vi "Set Debug Mode.vi"(8 "error in (no error)":errorcluster, 10 "debug":bool, 11 "path-with-auto-complete in":refnum<class "path-with-auto-complete.lvclass">) -> (0 "error out":errorcluster, 3 "path-with-auto-complete out":refnum<class "path-with-auto-complete.lvclass">)   [LabVIEW 2020, in "path-with-auto-complete.lvclass"]
doc: "The <b>Load State Data VI</b> is a dynamic dispatch VI that must be overwritten in every QControl Class that uses the State Data. If used it must <b>Call Parent Method</b>. This recursively loads the Data Value Reference to the data space for the QControl Class up the inheritance hierarchy that uses the Data Value Reference.\n<b> </b> <b> </b>\n©2016 Q Software Innovations, LLC (QSI)\nwritten by Quentin Alldredge\nproduced in LabVIEW 2015\n\nsupport@qsoftwareinnovations.com\nwww.qsoftwareinnovations.com\n\nAll rights reserved.\n\nRedistribution and use in source and binary forms, with or without modification, are permitted provided that the following conditions are met:\n\n * Redistributions of source code must retain the above copyright notice, this list of conditions and the following disclaimer.\n * Redistributions in binary form must reproduce the above copyright notice, this list of conditions and the following disclaimer in the documentation and/or other materials provided with the distribution.\n * Neither the name of Q Software Innovations, LLC. nor the names of its contributors may be used to endorse or promote products derived from this software without specific prior written permission.\n\nTHIS SOFTWARE IS PROVIDED BY THE COPYRIGHT HOLDERS AND CONTRIBUTORS \"AS IS\" AND ANY EXPRESS OR IMPLIED WARRANTIES, INCLUDING, BUT NOT LIMITED TO, THE IMPLIED WARRANTIES OF MERCHANTABILITY AND FITNESS FOR A PARTICULAR PURPOSE ARE DISCLAIMED. IN NO EVENT SHALL THE COPYRIGHT OWNER OR CONTRIBUTORS BE LIABLE FOR ANY DIRECT, INDIRECT, INCIDENTAL, SPECIAL, EXEMPLARY, OR CONSEQUENTIAL DAMAGES (INCLUDING, BUT NOT LIMITED TO, PROCUREMENT OF SUBSTITUTE GOODS OR SERVICES; LOSS OF USE, DATA, OR PROFITS; OR BUSINESS INTERRUPTION) HOWEVER CAUSED AND ON ANY THEORY OF LIABILITY, WHETHER IN CONTRACT, STRICT LIABILITY, OR TORT (INCLUDING NEGLIGENCE OR OTHERWISE) ARISING IN ANY WAY OUT OF THE USE OF THIS SOFTWARE, EVEN IF ADVISED OF THE POSSIBILITY OF SUCH DAMAGE."
uses:
  path-with-auto-complete.lvclass
  path-with-auto-complete.lvclass/path-with-auto-complete.ctl
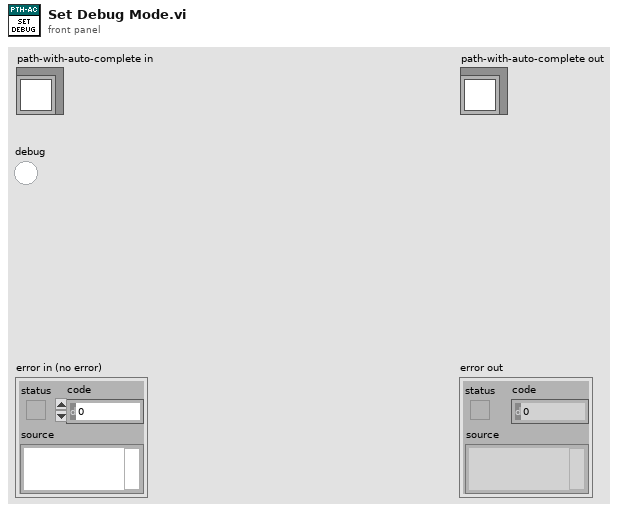
[diagram p1: front panel]
types:
  T1 = typedef "path-with-auto-complete.lvclass/State Data.ctl" = cluster{"Data":bool, "debug":bool, "mouse-down":bool, "has-focus":bool}
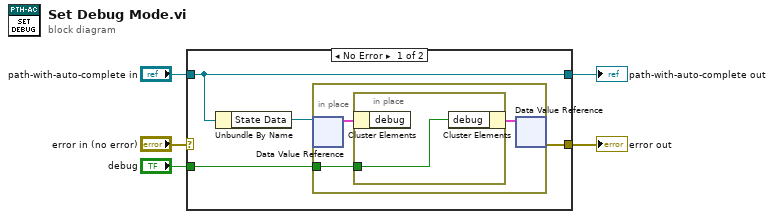
[diagram p0: block diagram]
diagram:
  n1 = case shown="No Error" "error in (no error)" {
    selector: "error in (no error)" -> [_ w15]
    tunnel: [w9 w15] -> w4
    tunnel: [w8 w14] -> w3
    tunnel: "path-with-auto-complete in" -> [w8 w14]
    tunnel: "debug" -> [w6 _]
    frame No Error {
      n2 = Unbundle By Name(w8) -> ("State Data"=w7:refnum<data-value>)
      n3 = in-place {
        in-place-border: w6 -> [w10]
        n4 = in-place-dvr #1(w7) -> (w12:T1)  [unwired: 1 out]
        n5 = in-place {
          in-place-border: w10 -> [w13]
          n6 = in-place-cluster #2(w12) -> ()  [unwired: 1 out]
          n7 = in-place-cluster #2("debug"=w13) -> (w11:T1)
        }
        n8 = in-place-dvr #1(w11) -> (w9:errorcluster)  [unwired: 1 out]
      }
    }
    frame Error {
    }
  }
  "error out" <- w4
  "path-with-auto-complete out" <- w3
